vi "Get VI Info Index by Name.vi"(8 "error in":errorcluster, 10 "VI name":string, 11 "state in":T1) -> (0 "error out":errorcluster, 1 "found?":bool, 2 "VI info index":i32, 3 "state out":T1)   [LabVIEW 2010, in "NI_SE_Config Front Panel Layout.lvlib"]
uses:
  NI_SE_Config Front Panel Layout.lvlib
  State.ctl
  VI Info.ctl
  VI Panel Layout/VI Panel Layout.lvclass
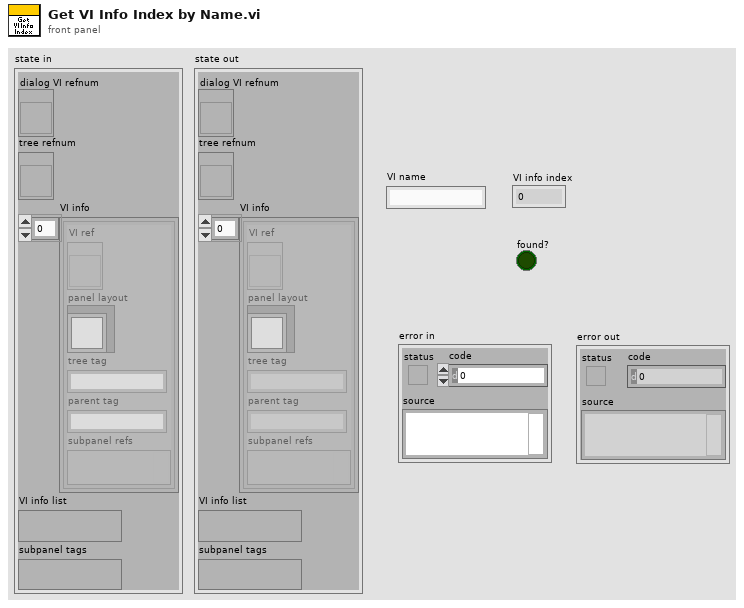
[diagram p1: front panel]
types:
  T1 = typedef "NI_SE_Config Front Panel Layout.lvlib/State.ctl" = cluster{"dialog VI refnum":refnum<vi>, "tree refnum":refnum<vi>, "VI info":T2[], "VI info list":variant, "subpanel tags":variant}
  T2 = typedef "NI_SE_Config Front Panel Layout.lvlib/VI Info.ctl" = cluster{"VI ref":refnum<vi>, "panel layout":refnum<class "VI Panel Layout.lvclass">, "tree tag":string, "parent tag":string, "subpanel refs":variant}
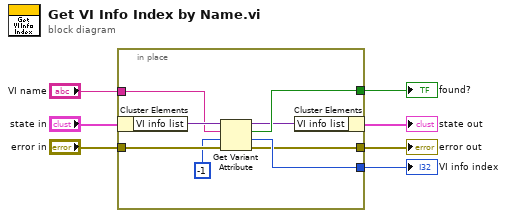
[diagram p0: block diagram]
diagram:
  n1 = in-place {
    in-place-border: "VI name" -> [w10]
    in-place-border: "error in" -> [w14]
    in-place-border: [w12] -> w2
    in-place-border: [w11] -> w6
    in-place-border: [w9] -> w1
    n2 = in-place-cluster #1("state in") -> ("VI info list"=w15:variant)
    n3 = Get Variant Attribute(Variant=w15, name=w10, default value (empty Variant)=-1, error in=w14) -> (duplicate Variant=w8:variant, found=w9:bool, value=w12:i32, error out=w11:errorcluster)
    n4 = in-place-cluster #1("VI info list"=w8) -> (→"state out":T1)
  }
  "error out" <- w6
  "VI info index" <- w2
  "found?" <- w1
